vi "WriteOpticalSwitch.vi"(4 "Output":i32, 6 "Input":i32, 11 "DAQ Port":tag) -> ()   [LabVIEW 2011]
uses:
  <vilib>/DAQmx/write.llb/DAQmx Write (Digital 1D Bool 1Chan 1Samp).vi
  <vilib>/DAQmx/create/channels.llb/DAQmx Create Channel (DO-Digital Output).vi
  <vilib>/DAQmx/miscellaneous.llb/DAQmx Fill In Error Info.vi
  Program Files (x86)/National Instruments/LabVIEW 2011/resource/objmgr/daqmx.rc
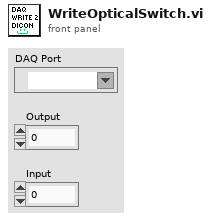
[diagram p1: front panel]
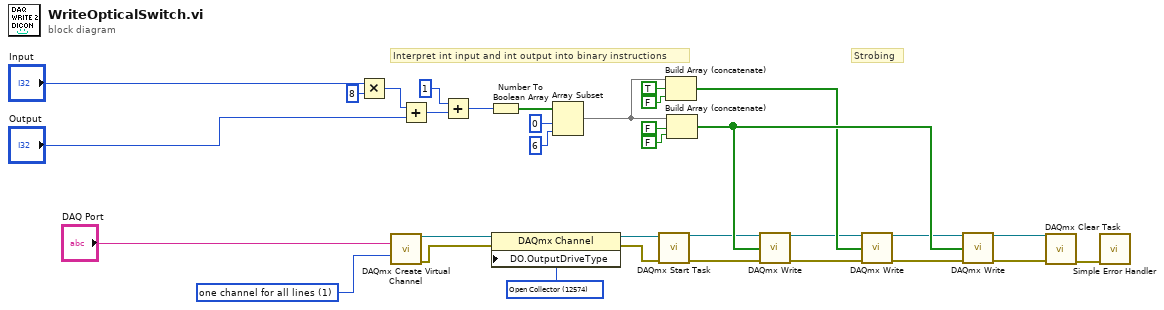
[diagram p0: block diagram]
diagram:
  w2 = 12574 items=["Active Drive"=12573, "Open Collector"=12574] ("DO.OutputDriveType")
  w3 = 1 items=["one channel for each line", "one channel for all lines"] ("line grouping")
  # "Strobing"
  # "Interpret int input and int output into binary instructions"
  n1 = Multiply(x="Input", y=8) -> (x*y=w17:i32)
  n2 = call-poly <vilib>:"DAQmx Create Virtual Channel.vi"("lines"="DAQ Port", "line grouping"=w3) -> ("task out"=w5:refnum<k21>, "error out"=w6:errorcluster)  [unwired: 12 in]
  n3 = Add(x=w17, y="Output") -> (x+y=w18:i32)
  n4 = Add(x=1, y=w18) -> (x+y=w19:i32)
  n5 = Number To Boolean Array(number=w19) -> (Boolean array=w20:bool[])
  n6 = property class="DAQmx Channel"(reference=w5, error in=w6, "DO.OutputDriveType"=w2) -> (reference out=w7:refnum<k21>, error out=w8:errorcluster)
  n7 = Array Subset(array=w20, index=0, length=6) -> (w1:bool[])
  n8 = call <vilib>:"DAQmx Start Task.vi"("task/channels in"=w7, "error in"=w8) -> ("task out"=w9:refnum<k21>, "error out"=w10:errorcluster)  [unwired: 12 in]
  n9 = Build Array (concatenate)(w1, TRUE, FALSE) -> (w27:bool[])
  n10 = Build Array (concatenate)(w1, FALSE, FALSE) -> (w30:bool[])
  n11 = call-poly <vilib>:"DAQmx Write.vi"("task/channels in"=w9, "data"=w30, "error in"=w10) -> ("task out"=w11:refnum<k21>, "error out"=w12:errorcluster)  [unwired: 10 in, 1 out]
  n12 = call-poly <vilib>:"DAQmx Write.vi"("task/channels in"=w11, "data"=w27, "error in"=w12) -> ("task out"=w28:refnum<k21>, "error out"=w29:errorcluster)  [unwired: 10 in, 1 out]
  n13 = call-poly <vilib>:"DAQmx Write.vi"("task/channels in"=w28, "data"=w30, "error in"=w29) -> ("task out"=w31:refnum<k21>, "error out"=w32:errorcluster)  [unwired: 10 in, 1 out]
  n14 = call <vilib>:"DAQmx Clear Task.vi"("task in"=w31, "error in"=w32) -> ("error out"=w33:errorcluster)  [unwired: 13 in]
  n15 = call <vilib>:"Simple Error Handler.vi"("error in (no error)"=w33) -> ()  [unwired: 4 in, 5 out]
